vi "Initialize DI.vi"(0 "DAQNode Dict":T1, 5 "DI Channels":T2[](array[typedef]), 9 "DI TaskName":string, 11 "error in":errorcluster, 14 "Simulate":bool) -> (4 "DAQNode Dict out":T1, 6 "DI IONames":string[](array[string]), 8 "DI SchemNames":string[](array[string]), 10 "DAQmx Task DI":refnum<k21>, 15 "error out":errorcluster)   [LabVIEW 2017, in "DAQ.lvclass"]
doc: "Developed by Kevin Thompson\nkevin@thompsonengineering.net\n\nCopyright 2015\nThompson Engineering, LLC"
uses:
  DAQ.lvclass
  DataTypes/TD DI Channel--cluster.ctl
  <vilib>/TELLC/Dynamic CVT API/TD Dynamic CVT DVR--ref.ctl
  DataTypes/TD DI TaskIO.ctl
  <vilib>/DAQmx/create/channels.llb/DAQmx Create Channel (DI-Digital Input).vi
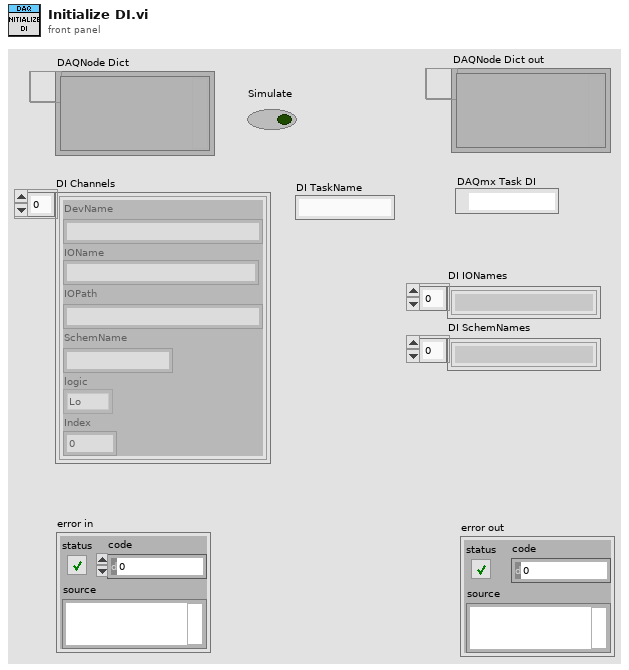
[diagram p1: front panel]
types:
  T1 = typedef "TD Dynamic CVT DVR--ref.ctl" = refnum<data-value>
  T2 = typedef "DAQ.lvclass/TD DI Channel--cluster.ctl" = cluster{"DevName":string, "IOName":string, "IOPath":string, "SchemName":string, "logic":enum16{"Lo", "Hi"}, "Index":i32}
  T3 = typedef "DAQ.lvclass/TD DI TaskIO.ctl" = cluster{"DI TaskName":string, "IONames":string[], "DAQmxDI TaskRef":refnum<k21>}
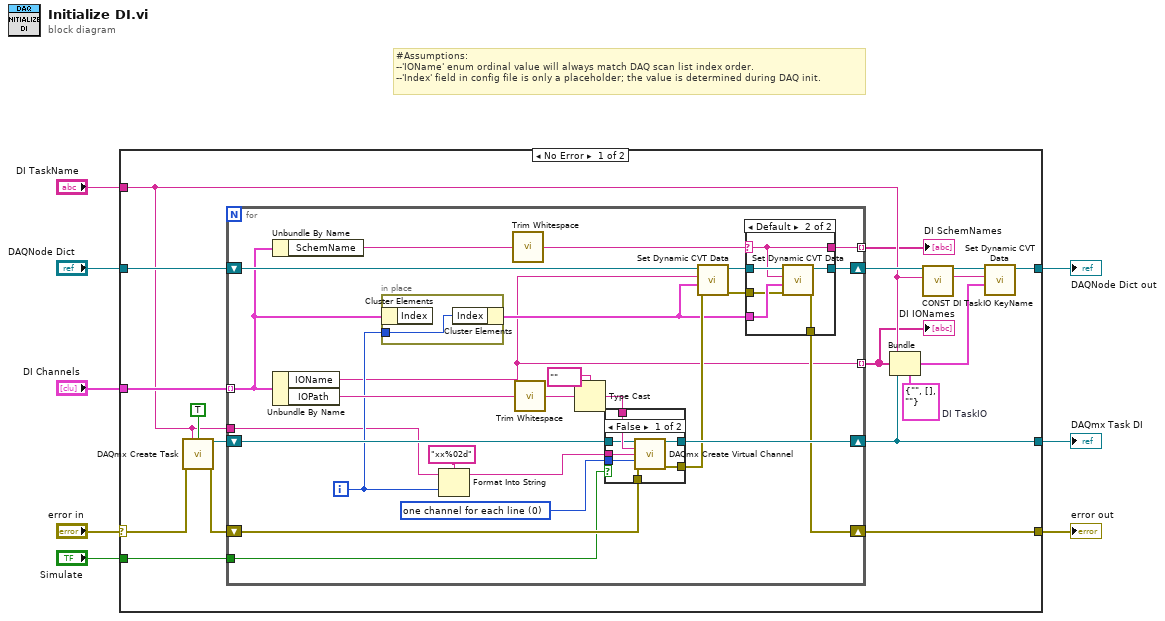
[diagram p0: block diagram]
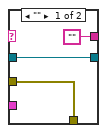
[diagram p2: hidden frame]
diagram:
  # "#Assumptions:\n--'IOName' enum ordinal value will always match DAQ scan list index order.\n--'Index' field in config file is only a placeholder; the value is determined during DAQ init."
  n1 = case shown="No Error" "error in" {
    selector: "error in" -> [w22 w71]
    tunnel: "DI Channels" -> [w19 _]
    tunnel: "DAQNode Dict" -> [w23 w70]
    tunnel: [w21 w71] -> w6
    tunnel: [w15 w70] -> w4
    tunnel: [w13 _] -> w3
    tunnel: "Simulate" -> [w9 _]
    tunnel: "DI TaskName" -> [w14 _]
    frame No Error {
      w12 = T3 {"DI TaskName"="", "IONames"=[], "DAQmxDI TaskRef"=""}  # DI TaskIO
      n2 = call <vilib>:"DAQmx Create Task.vi"("new task name"=w14, "auto cleanup"=TRUE, "error in"=w22) -> ("task out"=w24:refnum<k21>, "error out"=w25:errorcluster)  [unwired: 11 in]
      n3 = for {
        tunnel: w19 -> [w31] mode=indexing
        shift-right: [w35] -> w21
        shift-left: w25 -> [w42]
        shift-right: [w38] -> w16
        shift-left: w23 -> [w45]
        shift-right: [w43] -> w13
        shift-left: w24 -> [w44]
        tunnel: w14 -> [w29]
        tunnel: [w28] -> w10 mode=indexing
        tunnel: [w27] -> w11 mode=indexing
        tunnel: w9 -> [w26]
        i -> [w30]
        w40 = 0 items=["one channel for each line", "one channel for all lines"] ("line grouping")
        n4 = Unbundle By Name(w31) -> ("SchemName"=w37:string)
        n5 = Unbundle By Name(w31) -> ("IOName"=w28:string, "IOPath"=w50:string)
        n6 = in-place {
          in-place-border: w30 -> [w51]
          n7 = in-place-cluster #1(w31) -> ()  [unwired: 1 out]
          n8 = in-place-cluster #1("Index"=w51) -> (w32:T2)
        }
        n9 = Format Into String(format string="xx%02d", initial string=w29, w30) -> (resulting string=w46:string)  [unwired: 1 in, 1 out]
        n10 = call <vilib>:"Trim Whitespace.vi"("string"=w37) -> ("trimmed string"=w33:string)  [unwired: 1 in]
        n11 = call <vilib>:"Trim Whitespace.vi"("string"=w50) -> ("trimmed string"=w48:string)  [unwired: 1 in]
        n12 = Type Cast(type=tag "" ("lines"), x=w48) -> (*(type *) &x=w49:tag)
        n13 = case shown="False" w26 {
          tunnel: w49 -> [w67 _]
          tunnel: w46 -> [w66 _]
          tunnel: w44 -> [w65 w69]
          tunnel: [w64 w69] -> w43
          tunnel: w42 -> [w63 w68]
          tunnel: w40 -> [w62 _]
          tunnel: [w61 w68] -> w34
          frame False {
            n14 = call-poly <vilib>:"DAQmx Create Virtual Channel.vi"("task in"=w65, "lines"=w67, "name to assign"=w66, "line grouping"=w62, "error in"=w63) -> ("task out"=w64:refnum<k21>, "error out"=w61:errorcluster)  [unwired: 9 in]
          }
          frame True {
          }
        }
        n15 = call <vilib>:"Set Dynamic CVT Data.vi"("error in (no error)"=w34, "value"=w32, "DataName"=w28, "dCVT DVR"=w45) -> ("error out"=w36:errorcluster, "dCVT DVR out"=w39:T1)  [unwired: 5 in, 1 out]
        n16 = case shown="Default" w33 {
          selector: w33 -> [_ w55]
          tunnel: w39 -> [w54 w60]
          tunnel: [w54 w59] -> w38
          tunnel: w32 -> [_ w58]
          tunnel: w36 -> [w53 w57]
          tunnel: [w53 w56] -> w35
          tunnel: ["" w55] -> w27
          frame "" {
          }
          frame Default {
            n17 = call <vilib>:"Set Dynamic CVT Data.vi"("error in (no error)"=w57, "value"=w58, "DataName"=w55, "dCVT DVR"=w60) -> ("error out"=w56:errorcluster, "dCVT DVR out"=w59:T1)  [unwired: 5 in, 1 out]
          }
        }
      }
      "DI SchemNames" <- w11
      "DI IONames" <- w10
      n18 = Bundle(cluster=w12, "DI TaskName"=w14, "IONames"=w10, "DAQmxDI TaskRef"=w13) -> (w17:T3)
      n19 = call "CONST DI TaskIO KeyName.vi"("DI TaskName"=w14) -> ("DI TaskIO (KeyName)"=w18:string)  [unwired: 10 in]
      n20 = call <vilib>:"Set Dynamic CVT Data.vi"("value"=w17, "DataName"=w18, "dCVT DVR"=w16) -> ("dCVT DVR out"=w15:T1)  [unwired: 6 in, 2 out]
    }
    frame Error {
    }
  }
  "error out" <- w6
  "DAQNode Dict out" <- w4
  "DAQmx Task DI" <- w3
